vi "Initialize Core.vi"(8 "error in (no error)":errorcluster, 10 "Parameters":refnum<class "Abstract Init Parameters.lvclass">, 11 "Abstract Consumer in":refnum<class "Abstract Consumer.lvclass">) -> (0 "error out":errorcluster, 3 "Abstract Consumer out":refnum<class "Abstract Consumer.lvclass">)   [LabVIEW 2027, in "Messaging.lvlib" / "Abstract Consumer.lvclass"]
uses:
  Abstract Consumer.lvclass
  Parameters/Abstract Init Parameters/Abstract Init Parameters.lvclass
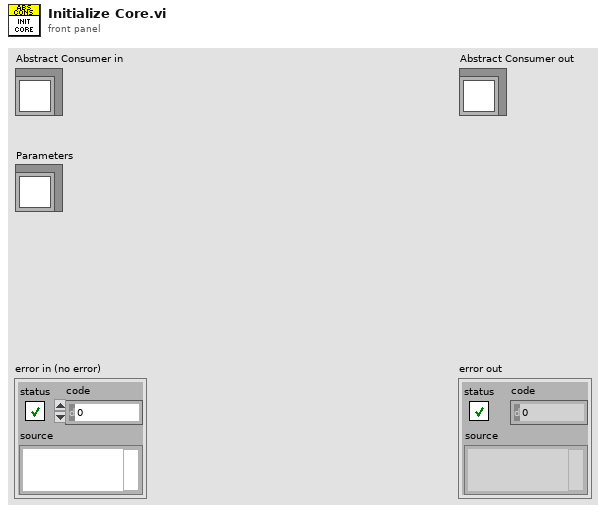
[diagram p1: front panel]
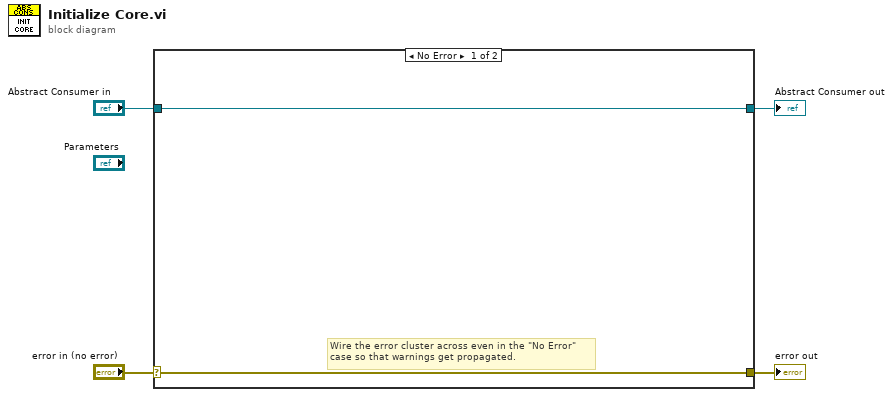
[diagram p0: block diagram]
diagram:
  n1 = case shown="No Error" "error in (no error)" {
    selector: "error in (no error)" -> [w5 w8]
    tunnel: [w5 w8] -> w3
    tunnel: [w6 w7] -> w1
    tunnel: "Abstract Consumer in" -> [w6 w7]
    frame No Error {
      # "Wire the error cluster across even in the \"No Error\"\ncase so that warnings get propagated."
    }
    frame Error {
    }
  }
  "error out" <- w3
  "Abstract Consumer out" <- w1
